vi "Send Message.vi"(6 "Event ID (None)":string, 7 "Event Name (None)":string, 8 "error in (no error)":errorcluster, 10 "Data":string, 11 "SSE Client in":refnum<class "SSE Client.lvclass">) -> (0 "error out":errorcluster, 3 "SSE Client out":refnum<class "SSE Client.lvclass">)   [LabVIEW 2020, in "HTTP Server.lvlib" / "SSE Client.lvclass"]
uses:
  SSE Client.lvclass
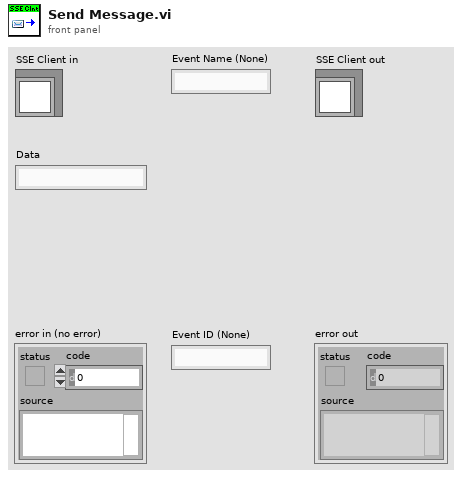
[diagram p1: front panel]
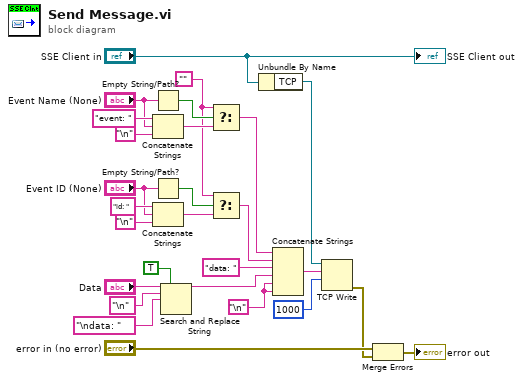
[diagram p0: block diagram]
diagram:
  w7 = "\n"
  w10 = ""
  n1 = Empty String/Path?(string/path="Event Name (None)") -> (empty?=w16:bool)
  n2 = Concatenate Strings("event: " ("string"), "Event Name (None)", "\n") -> (w17:string)
  n3 = Empty String/Path?(string/path="Event ID (None)") -> (empty?=w15:bool)
  n4 = Concatenate Strings("id: " ("string"), "Event ID (None)", "\n") -> (w14:string)
  n5 = Search and Replace String(replace all?=TRUE ("replace all? (F)"), input string="Data", search string="\n", replace string="\ndata: " ("search string")) -> (result string=w21:string)  [unwired: 4 in, 3 out]
  n6 = Select(t=w10, s=w16, f=w17) -> (s? t:f=w8:string)
  n7 = Select(t=w10, s=w15, f=w14) -> (s? t:f=w9:string)
  n8 = Unbundle By Name("SSE Client in") -> ("TCP"=w4:refnum<k5>)
  n9 = Concatenate Strings(w8, w9, "data: " ("string"), w21, w7, w7) -> (w5:string)
  n10 = TCP Write(connection ID=w4, data in=w5, 9:1000 ("timeout ms (25000)")) -> (error out=w1:errorcluster)  [unwired: 1 in, 2 out]
  n11 = Merge Errors("error in (no error)", w1) -> (→"error out":errorcluster)
  "SSE Client out" <- "SSE Client in"
